vi "FloderCreate.vi"(11 "Combo Box":string(combo)="BarcodeSetting") -> (3 "File Path":path[](array[path]))   [LabVIEW 2015]
uses:
  Galobal variable_TI.vi
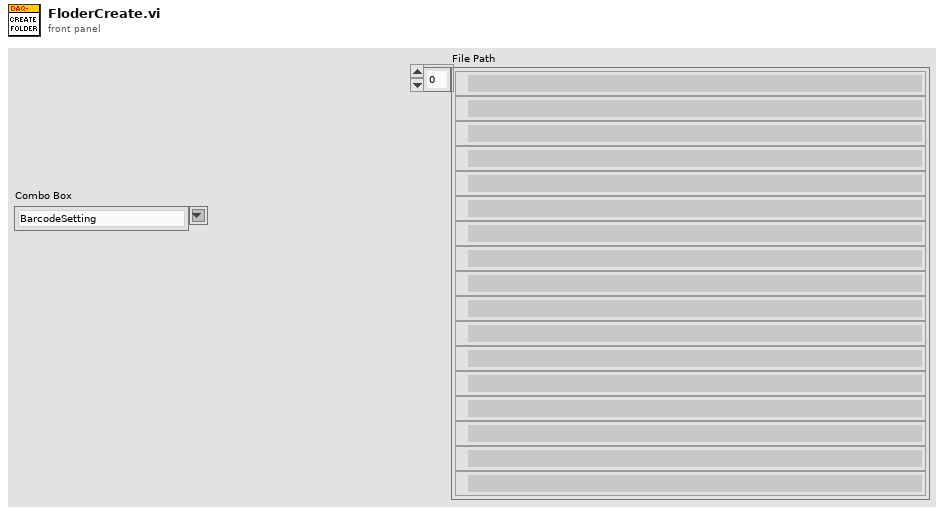
[diagram p1: front panel]
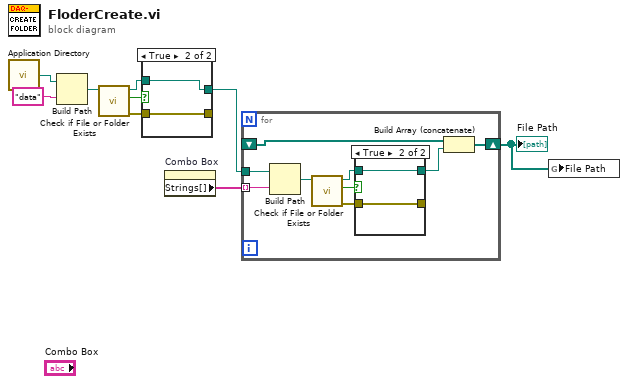
[diagram p0: block diagram]
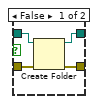
[diagram p2: hidden frame]
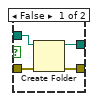
[diagram p3: hidden frame]
diagram:
  n1 = call <vilib>:"Application Directory.vi"() -> ("Application Directory"=w2:path)
  n2 = Build Path(base path=w2, name or relative path="data") -> (appended path=w8:path)
  n3 = call <vilib>:"Check if File or Folder Exists.vi"("path"=w8) -> ("error out"=w5:errorcluster, "file or folder exists?"=w7:bool, "dup path"=w6:path)  [unwired: 8 in]
  n4 = case shown="True" w7 {
    tunnel: w6 -> [w13 w15]
    tunnel: w5 -> [w12 w14]
    tunnel: [w11 w15] -> w4
    tunnel: [w10 w14] -> _
    frame False {
      n5 = Create Folder(path (use dialog)=w13, error in=w12) -> (created path=w11:path, error out=w10:errorcluster)  [unwired: 1 in, 1 out]
    }
    frame True {
    }
  }
  n6 = property on="Combo Box" class="CmbBox"() -> ("Strings[]"=w3:string[])  [unwired: 2 in, 2 out]
  n7 = for {
    tunnel: w4 -> [w20]
    tunnel: w3 -> [w19] mode=indexing
    shift-right: [w17] -> w1
    shift-left: _ -> [w16]
    n8 = Build Path(base path=w20, name or relative path=w19) -> (appended path=w21:path)
    n9 = call <vilib>:"Check if File or Folder Exists.vi"("path"=w21) -> ("error out"=w24:errorcluster, "file or folder exists?"=w22:bool, "dup path"=w23:path)  [unwired: 8 in]
    n10 = case shown="True" w22 {
      tunnel: w23 -> [w28 w30]
      tunnel: w24 -> [w27 w29]
      tunnel: [w26 w30] -> w18
      tunnel: [w25 w29] -> _
      frame False {
        n11 = Create Folder(path (use dialog)=w28, error in=w27) -> (created path=w26:path, error out=w25:errorcluster)  [unwired: 1 in, 1 out]
      }
      frame True {
      }
    }
    n12 = Build Array (concatenate)(w16, w18) -> (w17:path[])
  }
  "File Path" <- w1
  n13 = global write "Galobal variable_TI.vi" "File Path"(w1) -> ()
